vi "Desired_Pos_Highligthing_1.vi"(7 "[IN] Thickness":i32, 8 "error IN":errorcluster, 10 "[IN] ROI":T2, 11 "[IN] Image":T1) -> (0 "error OUT":errorcluster)   [LabVIEW 2020]
uses:
  <vilib>/vision/Image Controls.llb/IMAQ Image.ctl
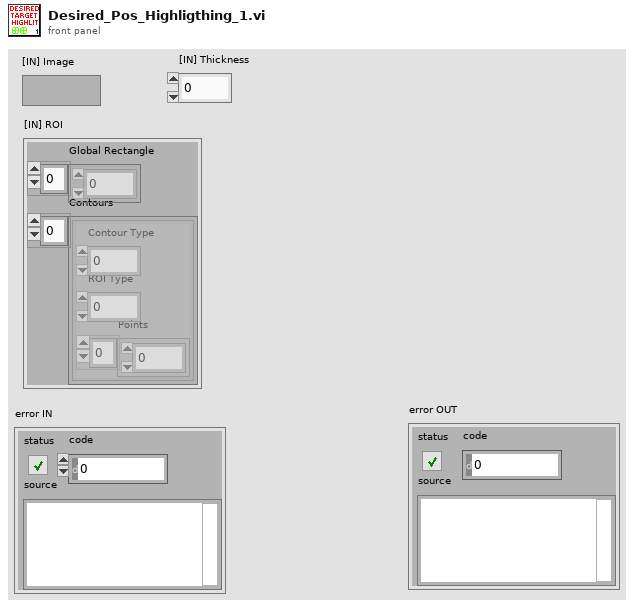
[diagram p1: front panel]
types:
  T1 = typedef "IMAQ Image.ctl" = refnum<image>
  T2 = cluster{"Global Rectangle":i32[], "Contours":cluster{"Contour Type":u32, "ROI Type":u32, "Points":i32[]}[]}
  T3 = cluster{"Contour Type":u32, "ROI Type":u32, "Points":i32[]}[]
  T4 = cluster{"Left":i32, "Top":i32, "Right":i32, "Bottom":i32}
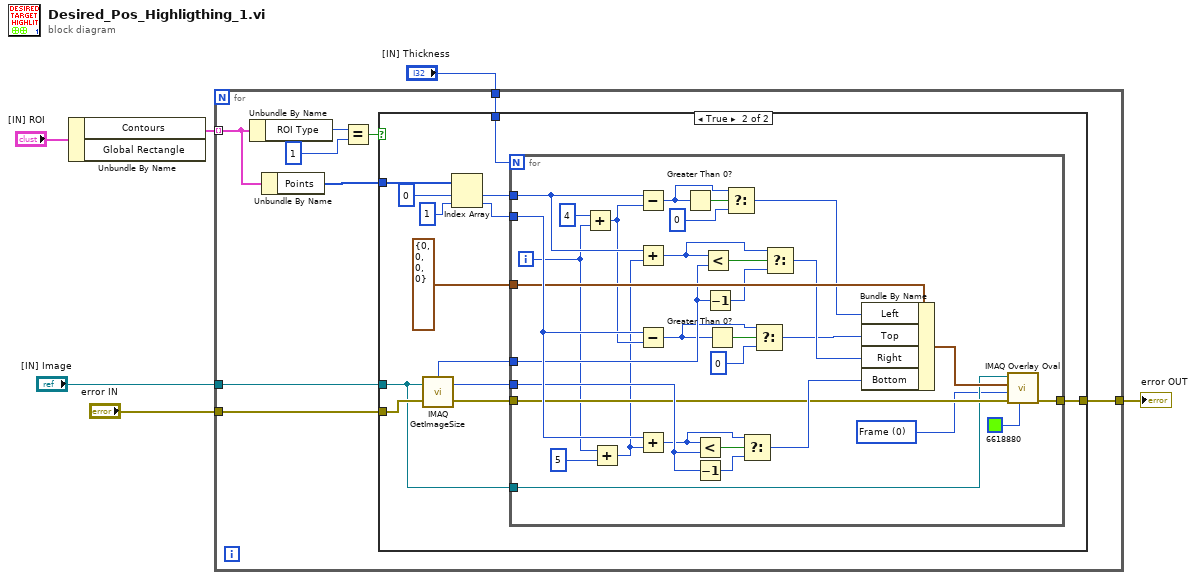
[diagram p0: block diagram]
diagram:
  n1 = Unbundle By Name("[IN] ROI") -> ("Contours"=w5:T3)  [unwired: 1 out]
  n2 = for {
    tunnel: w5 -> [w12] mode=indexing
    tunnel: "[IN] Image" -> [w10]
    tunnel: "error IN" -> [w9]
    tunnel: [w8] -> w2
    tunnel: "[IN] Thickness" -> [w7]
    n3 = Unbundle By Name(w12) -> ("ROI Type"=w15:u32)
    n4 = Unbundle By Name(w12) -> ("Points"=w11:i32[])
    n5 = Equal?(x=w15, y=u32 1) -> (x = y?=w13:bool)
    n6 = case shown="True" w13 {
      tunnel: w11 -> [_ w29]
      tunnel: w10 -> [_ w19]
      tunnel: w9 -> [w16 w23]
      tunnel: [w16 w18] -> w8
      tunnel: w7 -> [_ w17]
      frame False {
      }
      frame True {
        n7 = call "IMAQ GetImageSize"("Image"=w19, "error in (no error)"=w23) -> ("Y Resolution"=w21:i32, "X Resolution"=w22:i32, "error out"=w20:errorcluster)  [unwired: 2 in]
        n8 = Index Array(array=w29, index #1=0 ("index"), index #2=1 ("index")) -> (element #1=w26:i32, element #2=w25:i32)
        n9 = for {
          N: w17 -> [_]
          tunnel: w26 -> [w61]
          tunnel: w25 -> [w60]
          tunnel: T4 {"Left"=0, "Top"=0, "Right"=0, "Bottom"=0} ("Bounding Rectangle") -> [w56]
          tunnel: w22 -> [w53]
          tunnel: w21 -> [w44]
          tunnel: w19 -> [w38]
          tunnel: w20 -> [w40]
          tunnel: [w36] -> w18
          i -> [w31]
          w35 = u32 0 items=["Frame", "Fill"] ("Drawing Mode (Frame)")
          n10 = Add(x=4 ("y"), y=w31) -> (x+y=w33:i32)
          n11 = Add(x=w31, y=5) -> (x+y=w30:i32)
          n12 = Subtract(x=w61, y=w33) -> (x-y=w58:i32)
          n13 = Add(x=w61, y=w30) -> (x+y=w54:i32)
          n14 = Subtract(x=w60, y=w33) -> (x-y=w48:i32)
          n15 = Add(x=w60, y=w30) -> (x+y=w43:i32)
          n16 = Greater Than 0?(x=w58) -> (x > 0?=w59:bool)
          n17 = Less?(x=w43, y=w44) -> (x < y?=w45:bool)
          n18 = Decrement(x=w44) -> (x-1=w42:i32)
          n19 = Less?(x=w54, y=w53) -> (x < y?=w55:bool)
          n20 = Decrement(x=w53) -> (x-1=w52:i32)
          n21 = Greater Than 0?(x=w48) -> (x > 0?=w49:bool)
          n22 = Select(t=w58, s=w59, f=0) -> (s? t:f=w51:i32)
          n23 = Select(t=w43, s=w45, f=w42) -> (s? t:f=w41:i32)
          n24 = Select(t=w48, s=w49, f=0) -> (s? t:f=w47:i32)
          n25 = Select(t=w54, s=w55, f=w52) -> (s? t:f=w50:i32)
          n26 = Bundle By Name(cluster=w56, "Left"=w51, "Top"=w47, "Right"=w50, "Bottom"=w41) -> (w39:T4)
          n27 = call "IMAQ Overlay Oval"("Color"=u32 6618880, "error in (no error)"=w40, "Drawing Mode (Frame)"=w35, "Bounding Rectangle"=w39, "Image"=w38) -> ("error out"=w36:errorcluster)  [unwired: 5 in, 1 out]
        }
      }
    }
  }
  "error OUT" <- w2
